vi "Add class.vi"() -> ()   [LabVIEW 2017, in "Error.lvlib"]
uses:
  Error.lvlib
  <vilib>/Utility/config.llb/Write Key (Boolean).vi
  <vilib>/Utility/config.llb/Write Key (String).vi
  <vilib>/Utility/config.llb/NI_LVConfig.lvlib
panel:
  out "Old?":bool
  in  "Info":string
  in  "Log":bool
  in  "Kill":bool
  in  "Code":i32
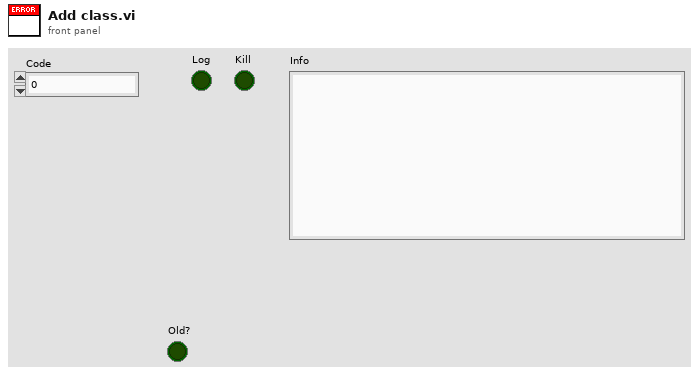
[diagram p1: front panel]
types:
  T1 = typedef "NI_LVConfig.lvlib/Config Data RefNum.ctl" = refnum<k1>
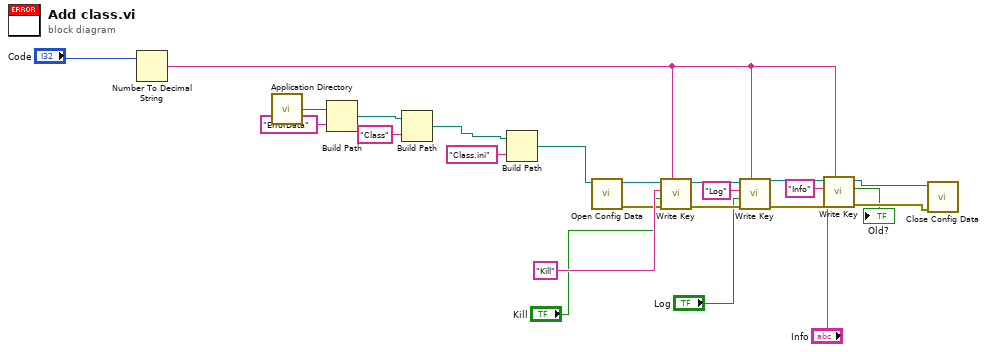
[diagram p0: block diagram]
diagram:
  n1 = Number To Decimal String(number="Code") -> (decimal integer string=w7:string)  [unwired: 1 in]
  n2 = call <vilib>:"Application Directory.vi"() -> ("Application Directory"=w23:path)
  n3 = Build Path(base path=w23, name or relative path="ErrorData") -> (appended path=w21:path)
  n4 = Build Path(base path=w21, name or relative path="Class") -> (appended path=w18:path)
  n5 = Build Path(base path=w18, name or relative path="Class.ini") -> (appended path=w17:path)
  n6 = call <vilib>:"Open Config Data.vi"("configuration file path"=w17) -> ("error out"=w13:errorcluster, "refnum"=w16:T1)  [unwired: 8 in, 1 out]
  n7 = call-poly <vilib>:"Write Key.vi"("section"=w7, "error in (no error)"=w13, "value"="Kill", "key"="Kill" ("name or relative path"), "refnum"=w16) -> ("error out"=w10:errorcluster, "refnum out"=w12:T1)  [unwired: 4 in, 1 out]
  n8 = call-poly <vilib>:"Write Key.vi"("section"=w7, "error in (no error)"=w10, "value"="Log", "key"="Log", "refnum"=w12) -> ("error out"=w9:errorcluster, "refnum out"=w8:T1)  [unwired: 4 in, 1 out]
  n9 = call-poly <vilib>:"Write Key.vi"("section"=w7, "error in (no error)"=w9, "value"="Info", "key"="Info", "refnum"=w8) -> ("error out"=w2:errorcluster, "found?"=→"Old?":bool, "refnum out"=w3:T1)  [unwired: 4 in]
  n10 = call <vilib>:"Close Config Data.vi"("error in (no error)"=w2, "refnum"=w3) -> ()  [unwired: 8 in, 2 out]
